vi "DSF.Memory.Buffer.Set Channel Count.vi"(8 "error in (no error)":errorcluster, 10 "channel count":u64 format="%d channels", 11 "Buffer in":refnum<class "DSF.Memory.Buffer.lvclass">) -> (0 "error out":errorcluster, 3 "Buffer out":refnum<class "DSF.Memory.Buffer.lvclass">)   [LabVIEW 2016, in "DSF.Memory.lvlib" / "DSF.Memory.Buffer.lvclass"]
uses:
  DSF.Memory.Buffer.lvclass
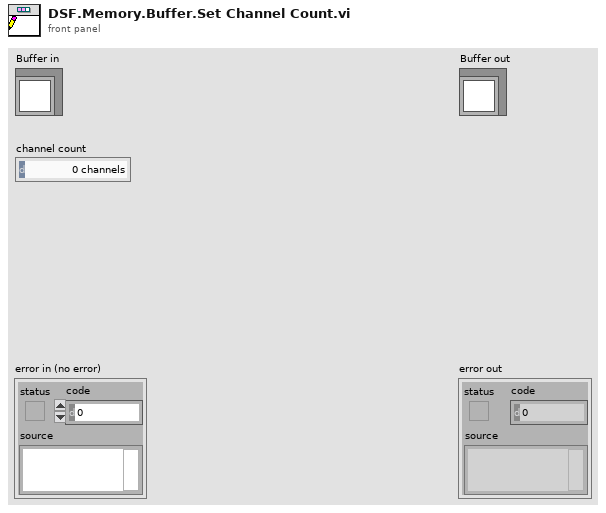
[diagram p1: front panel]
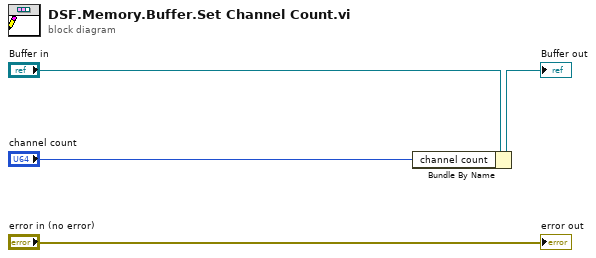
[diagram p0: block diagram]
diagram:
  n1 = Bundle By Name(cluster="Buffer in", "channel count"="channel count") -> (→"Buffer out":refnum<class "DSF.Memory.Buffer.lvclass">)
  "error out" <- "error in (no error)"
